vi "subVI_voltage_to_boolean.vi"(11 "voltage":dbl) -> (3 "binary":bool[](array[boolean]))   [LabVIEW 2019]
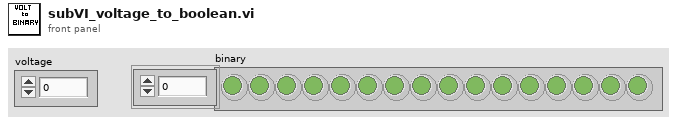
[diagram p1: front panel]
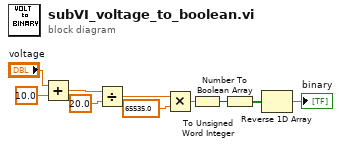
[diagram p0: block diagram]
diagram:
  n1 = Add(x="voltage", y=10.0) -> (x+y=w8:dbl)
  n2 = Divide(x=w8, y=20.0) -> (x/y=w4:dbl)
  n3 = Multiply(x=w4, y=65535.0) -> (x*y=w5:dbl)
  n4 = To Unsigned Word Integer(number=w5) -> (unsigned 16bit integer=w6:u16)
  n5 = Number To Boolean Array(number=w6) -> (Boolean array=w3:bool[])
  n6 = Reverse 1D Array(array=w3) -> (reversed array=→"binary":bool[])
